vi "setValue.vi"(8 "error in (no error)":errorcluster, 10 "value":variant, 11 "type.U8 in":refnum<class "type.DBL.lvclass">) -> (0 "error out":errorcluster, 3 "type.U8 out":refnum<class "type.DBL.lvclass">)   [LabVIEW 2015, in "type.DBL.lvclass"]
uses:
  type.DBL.lvclass
  type.DBL.lvclass/type.DBL.ctl
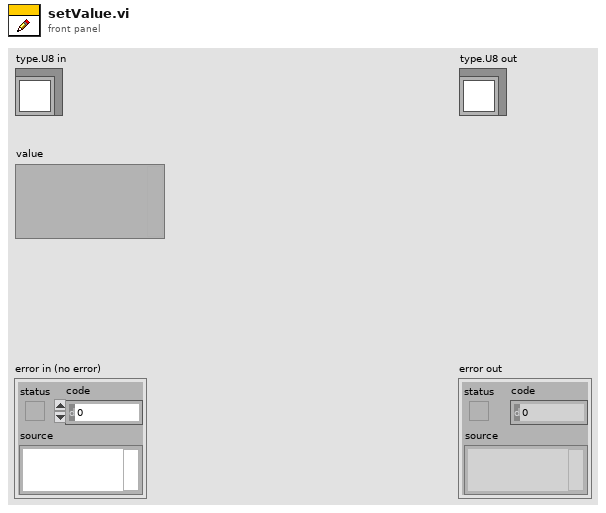
[diagram p1: front panel]
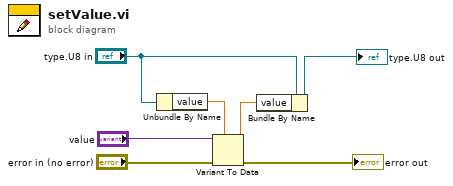
[diagram p0: block diagram]
diagram:
  n1 = Unbundle By Name("type.U8 in") -> ("value"=w4:dbl)
  n2 = Variant To Data(error in="error in (no error)", type=w4, Variant="value") -> (data=w3:dbl, error out=→"error out":errorcluster)
  n3 = Bundle By Name(cluster="type.U8 in", "value"=w3) -> (→"type.U8 out":refnum<class "type.DBL.lvclass">)
